vi "Pneumatics Config.vi"(8 "error in (no error)":errorcluster, 11 "Config in":refnum<class "Config.lvclass">) -> (0 "error out":errorcluster, 1 "IDs found?":bool, 2 "Pneumatics Data":T1, 3 "Config out":refnum<class "Config.lvclass">, 5 "File Found?":bool)   [LabVIEW 2019, in "Config.lvlib" / "Config.lvclass"]
doc: "Use this VI to get the IDs for the pneumatics of the robot."
uses:
  Config.lvclass
  Controls/Pneumatics Data.ctl
  <vilib>/Rock Robotics/WPI/Solenoid/WPI_SolenoidChannel.ctl
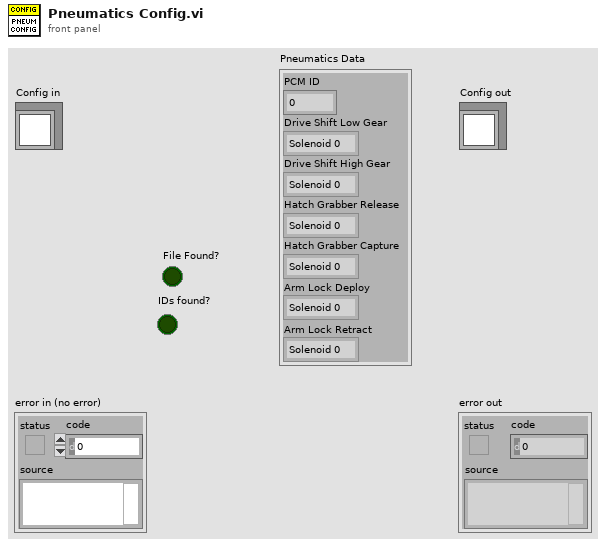
[diagram p1: front panel]
types:
  T1 = typedef "Config.lvlib/Config.lvclass/Pneumatics Data.ctl" = cluster{"PCM ID":u8, "Drive Shift Low Gear":T2, "Drive Shift High Gear":T2, "Hatch Grabber Release":T2, "Hatch Grabber Capture":T2, "Arm Lock Deploy":T2, "Arm Lock Retract":T2}
  T2 = typedef "WPI_SolenoidChannel.ctl" = enum8{"Solenoid 0", "Solenoid 1", "Solenoid 2", "Solenoid 3", "Solenoid 4", "Solenoid 5", "Solenoid 6", "Solenoid 7", "Invalid"}
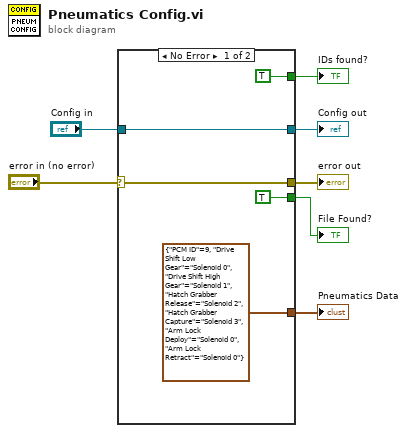
[diagram p0: block diagram]
diagram:
  n1 = case shown="No Error" "error in (no error)" {
    selector: "error in (no error)" -> [w11 w14]
    tunnel: [w11 w14] -> w6
    tunnel: [w12 w13] -> w4
    tunnel: "Config in" -> [w12 w13]
    tunnel: [TRUE ("IDs found?") _] -> w3
    tunnel: [TRUE ("File Found?") _] -> w2
    tunnel: [T1 {"PCM ID"=9, "Drive Shift Low Gear"=enum."Solenoid 0", "Drive Shift High Gear"=enum."Solenoid 1", "Hatch Grabber Release"=enum."Solenoid 2", "Hatch Grabber Capture"=enum."Solenoid 3", "Arm Lock Deploy"=enum."Solenoid 0", "Arm Lock Retract"=enum."Solenoid 0"} ("Pneumatics Data") _] -> w1
    frame No Error {
    }
    frame Error {
    }
  }
  "error out" <- w6
  "Config out" <- w4
  "File Found?" <- w2
  "IDs found?" <- w3
  "Pneumatics Data" <- w1
